vi "Make Connections (Parallel).vi"(8 "error in (no error)":errorcluster, 10 "switchActionsArray":T1 {"RelayAction" items=["CloseRelay"=21, "OpenRelay"=20]}, 11 "SLSC Switch in":refnum<class "SLSC Switch.lvclass">) -> (0 "error out":errorcluster, 3 "SLSC Switch out":refnum<class "SLSC Switch.lvclass">)   [LabVIEW 2015, in "SLSC Switch.lvlib" / "SLSC Switch.lvclass"]
uses:
  SLSC Switch.lvclass
  slscsl/SwitchActionsArray.ctl
  slscsl/SwitchAction.ctl
  slscsl/RelayAction.ctl
  SLSC Switch.lvclass/SLSC Switch.ctl
  Switch Action Processor/Switch Action Processor.lvclass
  slscsl/slscsl.lvclass
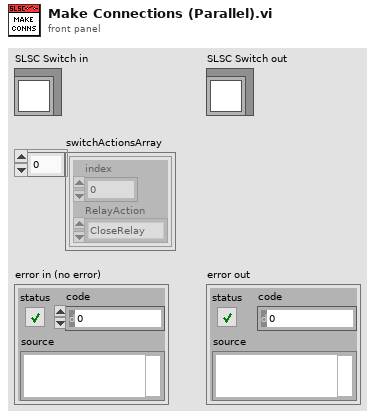
[diagram p1: front panel]
types:
  T1 = typedef "SLSC Switch.lvlib/slscsl.lvclass/SwitchActionsArray.ctl" = T2[]
  T2 = typedef "SLSC Switch.lvlib/slscsl.lvclass/SwitchAction.ctl" = cluster{"index":i32, "RelayAction":T3}
  T3 = typedef "SLSC Switch.lvlib/slscsl.lvclass/RelayAction.ctl" = u32
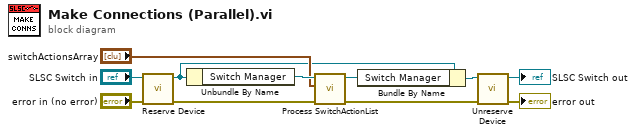
[diagram p0: block diagram]
diagram:
  n1 = call "Reserve Device.vi"("error in (no error)"="error in (no error)", "SLSC Switch in"="SLSC Switch in") -> ("error out"=w5:errorcluster, "SLSC Switch out"=w3:refnum<class "SLSC Switch.lvclass">)  [unwired: 8 in]
  n2 = Unbundle By Name(w3) -> ("Switch Manager"=w7:refnum<class "Switch Action Processor.lvclass">)
  n3 = call "Process SwitchActionList.vi"("error in (no error)"=w5, "SwitchActionList"="switchActionsArray", "Switch Action Processor In"=w7) -> ("error out"=w4:errorcluster, "Switch Action Processor Out"=w2:refnum<class "Switch Action Processor.lvclass">)  [unwired: 7 in]
  n4 = Bundle By Name(cluster=w3, "Switch Manager"=w2) -> (w1:refnum<class "SLSC Switch.lvclass">)
  n5 = call "Unreserve Device.vi"("error in (no error)"=w4, "SLSC Switch in"=w1) -> ("error out"=→"error out":errorcluster, "SLSC Switch out"=→"SLSC Switch out":refnum<class "SLSC Switch.lvclass">)  [unwired: 8 in]
